vi "irqTest.vi"   [LabVIEW 2016]
uses:
  <vilib>/rvi/Emulation/niFpgaGetClockAttributes.vi
  <vilib>/rvi/Emulation/niFpgaSctlEmulationGetInTimedLoop.vi
  <vilib>/rvi/Emulation/niFpgaEmulationReportErrorSimple.vi
  <vilib>/rvi/Emulation/niFpgaCriticalErrorInLSC.vi
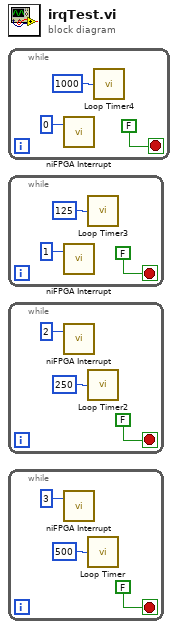
[diagram p0: block diagram]
diagram:
  n1 = while {
    stop <- FALSE stop-if-true
    n2 = call <vilib>:"niFPGA Interrupt.vi"("IRQ Number (0)"=u8 0) -> ()  [unwired: 2 in]
    n3 = call "Loop Timer4"("Count(mSec)"=u32 1000) -> ()  [unwired: 1 out]
  }
  n4 = while {
    stop <- FALSE stop-if-true
    n5 = call <vilib>:"niFPGA Interrupt.vi"("IRQ Number (0)"=u8 1) -> ()  [unwired: 2 in]
    n6 = call "Loop Timer3"("Count(mSec)"=u32 125) -> ()  [unwired: 1 out]
  }
  n7 = while {
    stop <- FALSE stop-if-true
    n8 = call <vilib>:"niFPGA Interrupt.vi"("IRQ Number (0)"=u8 2) -> ()  [unwired: 2 in]
    n9 = call "Loop Timer2"("Count(mSec)"=u32 250) -> ()  [unwired: 1 out]
  }
  n10 = while {
    stop <- FALSE stop-if-true
    n11 = call <vilib>:"niFPGA Interrupt.vi"("IRQ Number (0)"=u8 3) -> ()  [unwired: 2 in]
    n12 = call "Loop Timer"("Count(mSec)"=u32 500) -> ()  [unwired: 1 out]
  }
